vi "Shooter Simulator Reset Angle Encoder.vi"   [LabVIEW 2015]
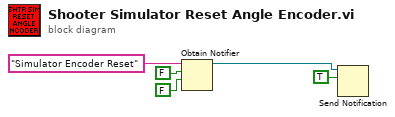
[diagram p0: block diagram]
diagram:
  n1 = Obtain Notifier(name (unnamed)="Simulator Encoder Reset", notification data type=FALSE, create if not found? (T)=FALSE) -> (notifier out=w2:refnum<notifier>)  [unwired: 1 in, 2 out]
  n2 = Send Notification(notification=TRUE, notifier=w2) -> ()  [unwired: 1 in, 2 out]
